vi "Create Vibration Data (SubVI).vi"(7 "data":waveform(dbl), 8 "Stop":bool, 9 "Time has Elapsed":bool, 10 "Cluster in":T2) -> (0 "Channel out":T1, 3 "Cluster out":T2)   [LabVIEW 2017]
uses:
  <extravilib>/ChannelInstances/Stream-wfm(dbl)/)Channel.ctl
  <extravilib>/ChannelInstances/Stream-wfm(dbl)/Write With Abort.vi
  <extravilib>/ChannelInstances/Stream-wfm(dbl)/Endpoint.vi
  <extravilib>/ChannelInstances/Stream-wfm(dbl)/)Channel.vi
  <resource>/ChannelSupport/_ChannelSupport/WaitIfNeeded.vi
  <extravilib>/ChannelInstances/Stream-wfm(dbl).lvlib
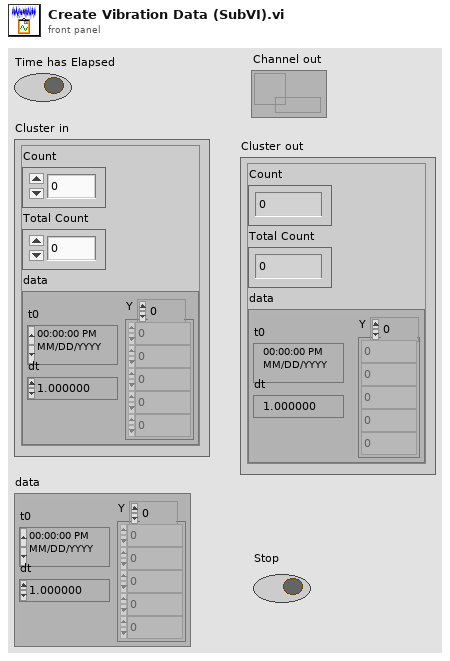
[diagram p1: front panel]
types:
  T1 = typedef "Stream-wfm(dbl).lvlib/)Channel.ctl" = refnum<queue>
  T2 = cluster{"Count":i32, "Total Count":dbl, "data":waveform(dbl)}
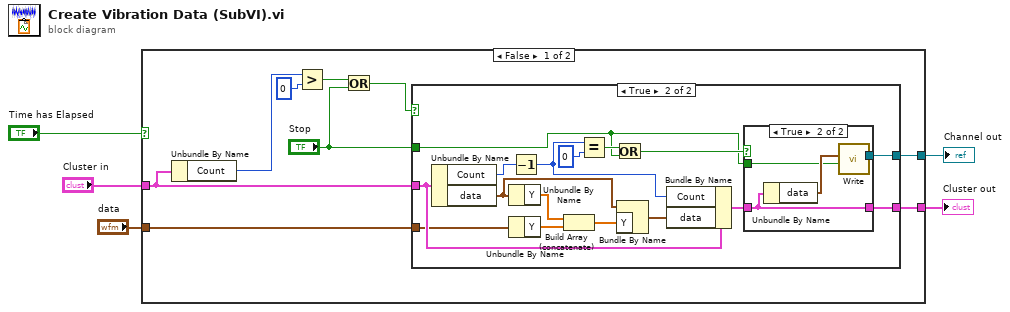
[diagram p0: block diagram]
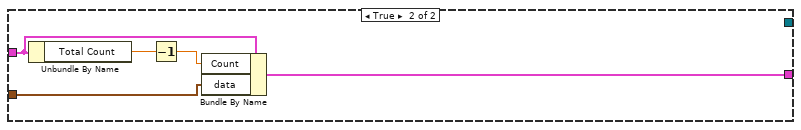
[diagram p4: hidden frame]
diagram:
  n1 = case shown="False" "Time has Elapsed" {
    tunnel: "data" -> [w11 w38]
    tunnel: "Cluster in" -> [w10 w40]
    tunnel: [w9 w39] -> w5
    tunnel: [w6 _] -> w1
    frame False {
      n2 = Unbundle By Name(w10) -> ("Count"=w14:i32)
      n3 = Greater?(x=w14, y=0) -> (0:w12:bool)
      n4 = Or(x=w12, y="Stop") -> (x .or. y?=w8:bool)
      n5 = case shown="True" w8 {
        tunnel: w11 -> [_ w19]
        tunnel: w10 -> [w15 w26]
        tunnel: [w15 w21] -> w9
        tunnel: "Stop" -> [_ w17]
        tunnel: [_ w16] -> w6
        frame False {
        }
        frame True {
          n6 = Unbundle By Name(w26) -> ("Count"=w31:i32, "data"=w20:waveform(dbl))
          n7 = Unbundle By Name(w20) -> ("Y"=w30:dbl[])
          n8 = Unbundle By Name(w19) -> ("Y"=w29:dbl[])
          n9 = Decrement(x=w31) -> (x-1=w25:i32)
          n10 = Build Array (concatenate)(w30, w29) -> (w28:dbl[])
          n11 = Equal?(x=w25, y=0) -> (x = y?=w23:bool)
          n12 = Or(x=w23, y=w17) -> (x .or. y?=w18:bool)
          n13 = Bundle By Name(cluster=w20, "Y"=w28) -> (w27:waveform(dbl))
          n14 = Bundle By Name(cluster=w26, "Count"=w25, "data"=w27) -> (w22:T2)
          n15 = case shown="True" w18 {
            tunnel: w22 -> [w32 w36]
            tunnel: [w32 w36] -> w21
            tunnel: w17 -> [_ w34]
            tunnel: [_ w33] -> w16
            frame False {
            }
            frame True {
              n16 = Unbundle By Name(w36) -> ("data"=w35:waveform(dbl))
              n17 = call <extravilib>:"Write.vi"("last element? (F)"=w34, "element"=w35) -> ("channel"=w33:T1)  [unwired: 7 in, 2 out]
            }
          }
        }
      }
    }
    frame True {
      n18 = Unbundle By Name(w40) -> ("Total Count"=w41:dbl)
      n19 = Decrement(x=w41) -> (x-1=w37:dbl)
      n20 = Bundle By Name(cluster=w40, "Count"=w37, "data"=w38) -> (w39:T2)
    }
  }
  "Cluster out" <- w5
  "Channel out" <- w1
